vi "Get Active Element Index.vi"(7 "Active Unique ID":string, 8 "error in (no error)":errorcluster, 10 "Active Test Executive Ref":refnum<data-value>, 11 "Test Executive Ref":refnum<data-value>) -> (0 "error out":errorcluster, 2 "Active Test Executive Ref out":refnum<data-value>, 3 "Test Executive Ref out":refnum<data-value>, 5 "Active Unique ID out":string)   [LabVIEW 2019, in "Test Executive.lvlib" / "TestExecutive Ref.lvclass"]
uses:
  <vilib>/gpm_packages/@cs/test-executive/Source/Test Executive/TestExecutive Ref/TestExecutive Ref.lvclass
  <vilib>/gpm_packages/@cs/test-executive/Source/Test Executive/ITestExecutive/ITest Executive.lvclass
  fb521218-5b40-4853-bd91-9f92150c73c1.vi
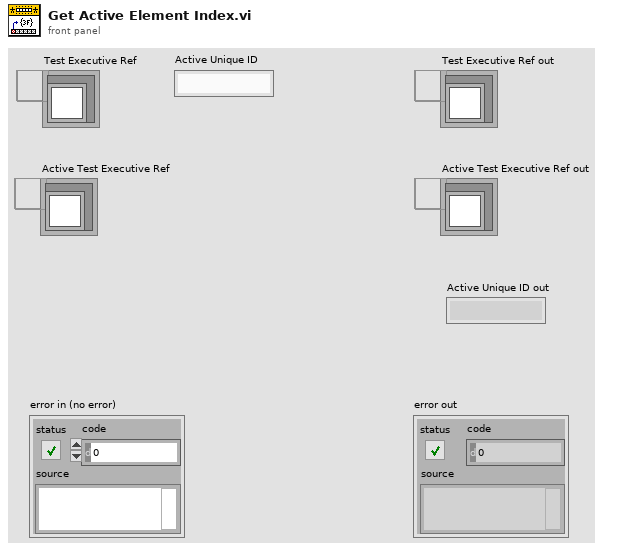
[diagram p1: front panel]
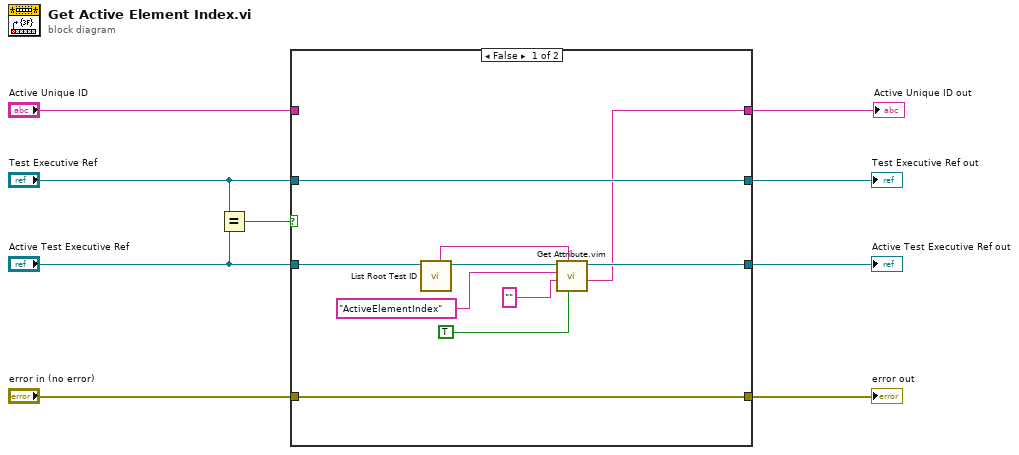
[diagram p0: block diagram]
diagram:
  n1 = Equal?(x="Test Executive Ref", y="Active Test Executive Ref") -> (x = y?=w2:bool)
  n2 = case shown="False" w2 {
    tunnel: "Test Executive Ref" -> [w19 w21]
    tunnel: "error in (no error)" -> [w10 w20]
    tunnel: "Active Test Executive Ref" -> [w11 w23]
    tunnel: [w17 w23] -> w8
    tunnel: [w19 w21] -> w7
    tunnel: "Active Unique ID" -> [_ w22]
    tunnel: [w10 w20] -> w5
    tunnel: [w12 w22] -> w1
    frame False {
      n3 = call <vilib>:"List Root Test ID.vi"("Test Executive Ref"=w11) -> ("Test Executive Ref out"=w18:refnum<data-value>, "Root ID"=w16:string)  [unwired: 6 in, 3 out]
      n4 = call "Get Attribute.vim"("Include Private?"=TRUE ("Private?"), "ID"=w16, "Type"="", "Attribute Name"="ActiveElementIndex", "Test Executive Ref"=w18) -> ("Attribute"=w12:string, "Test Executive Ref out"=w17:refnum<data-value>)  [unwired: 2 in, 3 out]
    }
    frame True {
    }
  }
  "Test Executive Ref out" <- w7
  "Active Test Executive Ref out" <- w8
  "error out" <- w5
  "Active Unique ID out" <- w1
